vi "enumerateStaticDependencies.vi"(8 "error in (no error)":errorcluster, 11 "SMO.D":refnum<class "SMO.D.lvclass">) -> (0 "error out":errorcluster, 2 "Static Dependencies":refnum<class "Dependency.lvclass">[](array[class]), 3 "SMO.D out":refnum<class "SMO.D.lvclass">)   [LabVIEW 2013, in "SMO.D.lvclass"]
uses:
  SMO.D.lvclass
  src/Dependency/Dependency.lvclass
  SMO.B/SMO.B.lvclass
  src/SMO/SMO.lvclass
panel:
  # "For instructions on how to use the JKI State Machine Objects, examples and video tutorials, visit:\nhttp://jki.net/state-machine-objects/\n\nJKI State Machine Objects™\nhttp://jki.net/state-machine-objects/\nCopyright (C) 2005-2015, JKI <info@jki.net>\nALL RIGHTS RESERVED"
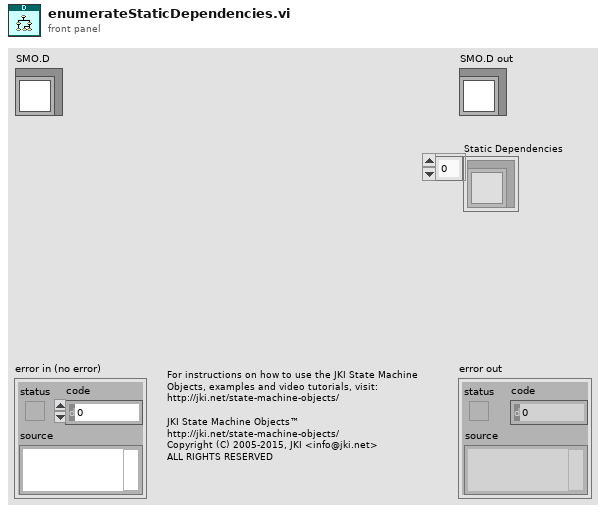
[diagram p1: front panel]
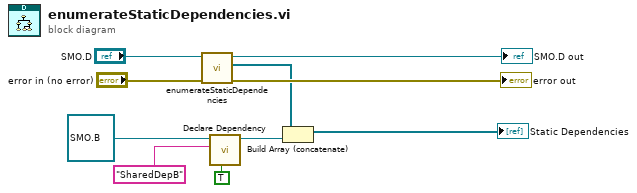
[diagram p0: block diagram]
diagram:
  n1 = call-parent "enumerateStaticDependencies.vi"("error in (no error)"="error in (no error)", "SMO"="SMO.D") -> ("error out"=→"error out":errorcluster, "Static Dependencies"=w3:refnum<class "Dependency.lvclass">[], "SMO out"=→"SMO.D out":refnum<class "SMO.D.lvclass">)  [unwired: 7 in]
  n2 = call "Declare Dependency.vi"("Shared Resource (F)"=TRUE, "Name"="SharedDepB", "Type"=refnum<class "SMO.B.lvclass"> refnum ("SMO.B.lvclass")) -> ("Dependency out"=w4:refnum<class "Dependency.lvclass">)  [unwired: 7 in, 1 out]
  n3 = Build Array (concatenate)(w3, w4) -> (→"Static Dependencies":refnum<class "Dependency.lvclass">[])
